vi "zad1_2.vi"() -> ()   [LabVIEW 2017]
uses:
  swiatla.ctl
panel:
  out "sygnalizator":T1
  in  "pause":bool
  in  "stop":bool
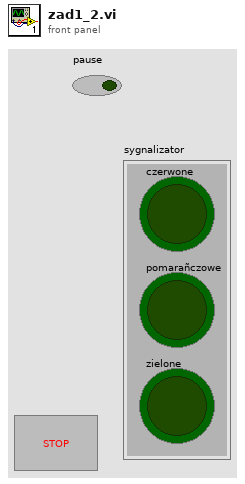
[diagram p1: front panel]
types:
  T1 = cluster{"czerwone":bool, "pomarañczowe":bool, "zielone":bool}
  T2 = typedef "swiatla.ctl" = enum16{"czerwone", "pomarañczowe", "zielone", "pomarañczowe i czerwone"}
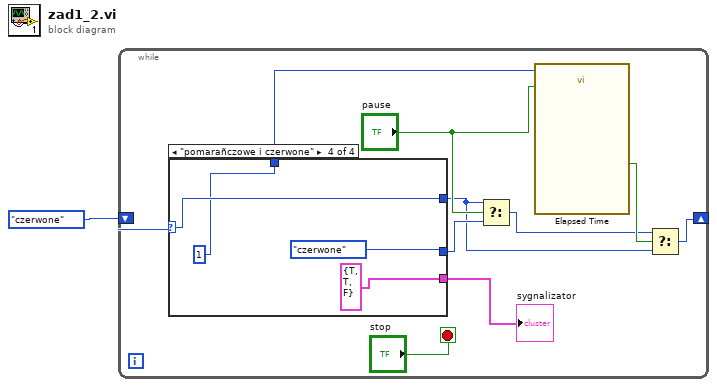
[diagram p0: block diagram]
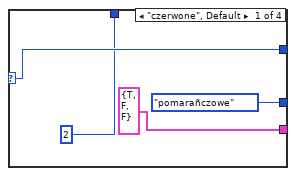
[diagram p2: hidden frame]
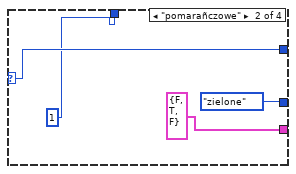
[diagram p3: hidden frame]
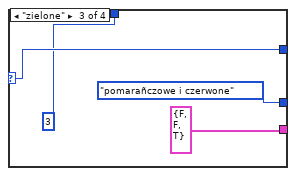
[diagram p4: hidden frame]
diagram:
  n1 = while {
    shift-right: [w6] -> _
    shift-left: swiatla."czerwone" -> [w11]
    stop <- "stop" stop-if-true
    n2 = case shown="\"pomarañczowe i czerwone\"" w11 {
      selector: w11 -> [w13 w17 w21 w26]
      tunnel: [T1 {"czerwone"=TRUE, "pomarañczowe"=FALSE, "zielone"=FALSE} ("sygnalizator") T1 {"czerwone"=FALSE, "pomarañczowe"=TRUE, "zielone"=FALSE} ("sygnalizator") T1 {"czerwone"=FALSE, "pomarañczowe"=FALSE, "zielone"=TRUE} ("sygnalizator") T1 {"czerwone"=TRUE, "pomarañczowe"=TRUE, "zielone"=FALSE} ("sygnalizator")] -> w9
      tunnel: [swiatla."pomarañczowe" swiatla."zielone" swiatla."pomarañczowe i czerwone" swiatla."czerwone"] -> w4
      tunnel: [w13 w17 w21 w26] -> w2
      tunnel: [u32 2 ("milliseconds to wait") u32 1 ("milliseconds to wait") u32 3 ("milliseconds to wait") u32 1 ("milliseconds to wait")] -> w8
      frame "czerwone", Default {
      }
      frame "pomarañczowe" {
      }
      frame "zielone" {
      }
      frame "pomarañczowe i czerwone" {
      }
    }
    "sygnalizator" <- w9
    n3 = Select(t=w2, s="pause", f=w4) -> (s? t:f=w3:T2)
    n4 = call "Elapsed Time"("Time Target (s)"=w8, "Reset"="pause") -> ("Time has Elapsed"=w7:bool)  [unwired: 10 in, 7 out]
    n5 = Select(t=w3, s=w7, f=w2) -> (s? t:f=w6:T2)
  }
